vi "Untitled 1.vi"() -> ()   [LabVIEW 2014]
uses:
  <vilib>/userdefined/High Color/IMAQdx.ctl
  <vilib>/vision/Classification.llb/IMAQ Classifier Session.ctl
  <vilib>/vision/driver/NI_Vision_Acquisition_Software.lvlib
  <resource>/objmgr/imaqdx.rc
panel:
  out "Boolean":bool
  out "Classes (Color Classification 1)":string[](array[string])
  out "Classifier Session (Color Classification 1)":T1
  in  "video mode":u32
  out "processed":T2(plugin-control)
  out "source":T2(plugin-control)
  in  "ESC":bool
  out "frame rate [fps]":dbl(slide) scale=0.0..30.0
  out "error out":errorcluster
  in  "webcam":T3="cam0"
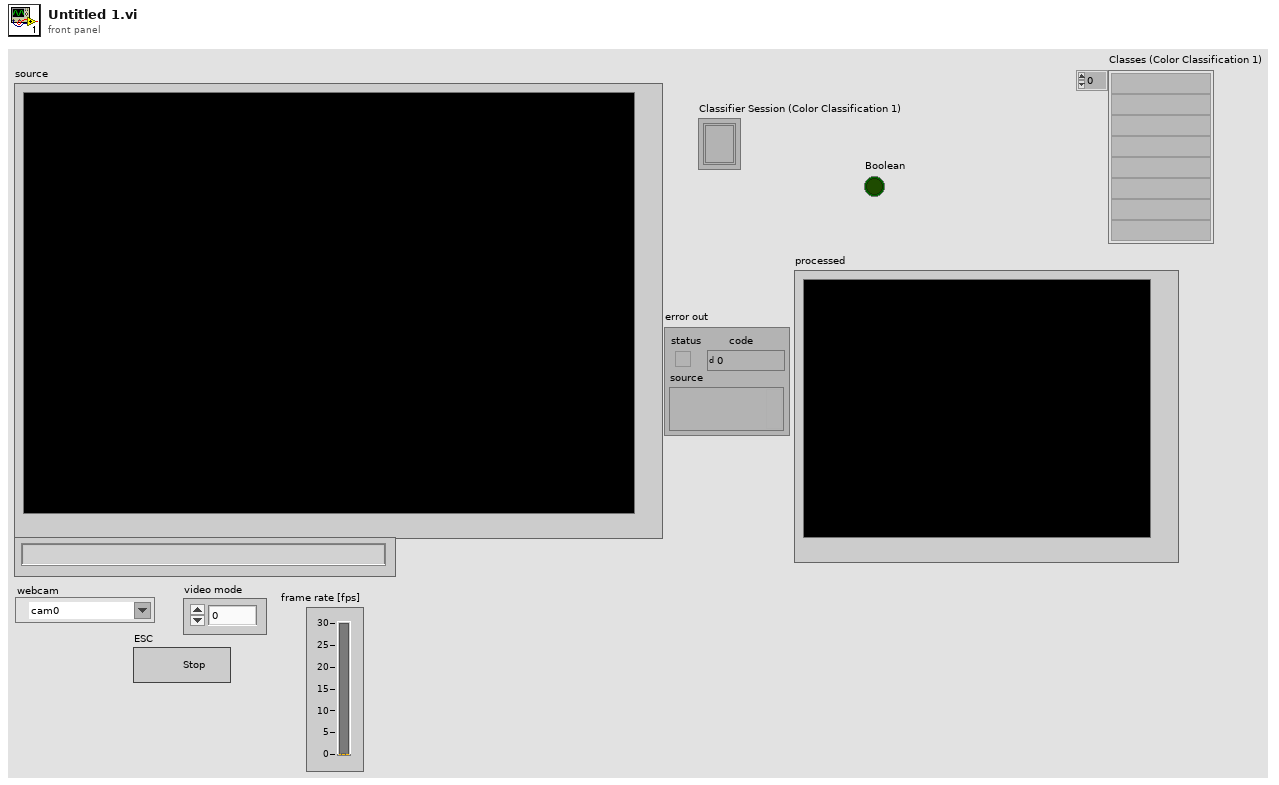
[diagram p1: front panel]
types:
  T1 = typedef "IMAQ Classifier Session.ctl" = refnum<k1>
  T2 = typedef "IMAQ Image.ctl" = refnum<image>
  T3 = typedef "IMAQdx.ctl" = refnum<k21>
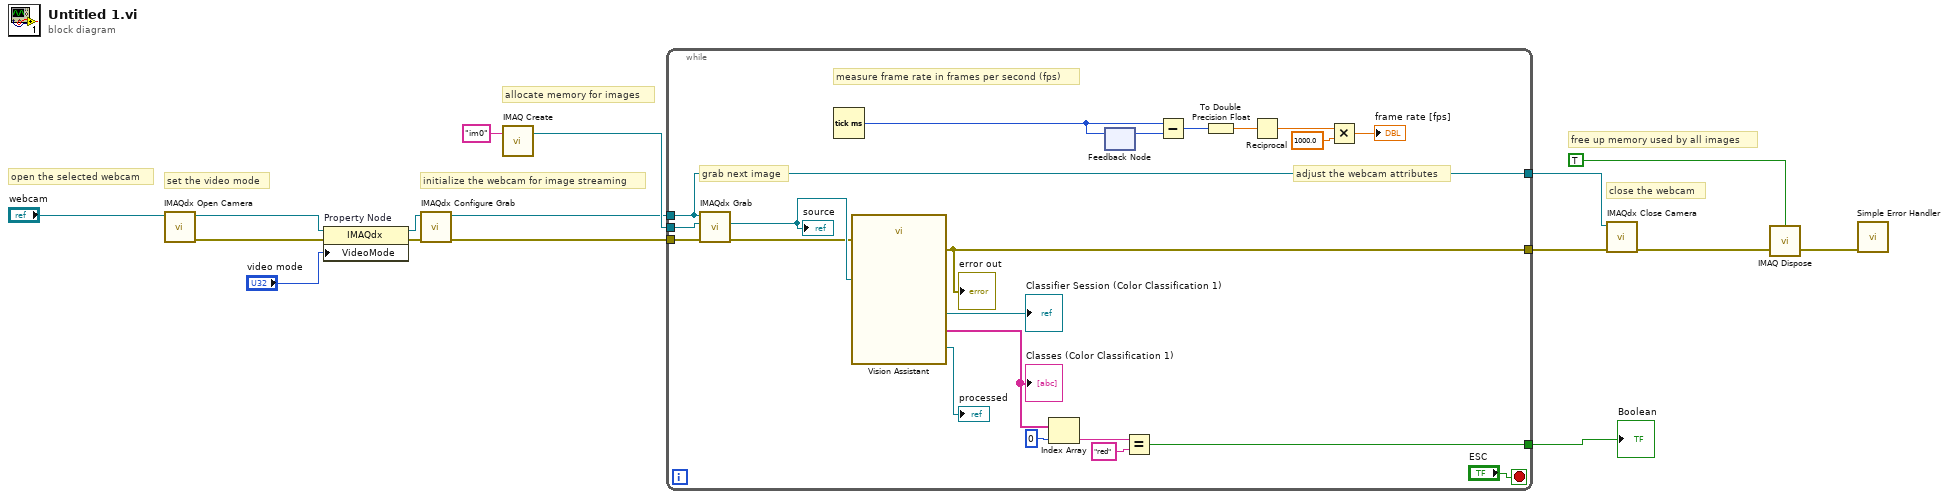
[diagram p0: block diagram]
diagram:
  # "close the webcam"
  # "open the selected webcam"
  # "set the video mode"
  # "allocate memory for images"
  # "initialize the webcam for image streaming"
  # "free up memory used by all images"
  n1 = call <vilib>:"IMAQdx Open Camera.vi"("Session In"="webcam") -> ("error out"=w7:errorcluster, "Session Out"=w6:T3)  [unwired: 2 in, 7 out]
  n2 = property on="Property Node" class="IMAQdx"(reference=w6, error in=w7, "VideoMode"="video mode") -> (reference out=w3:T3, error out=w4:errorcluster)
  n3 = call <vilib>:"IMAQdx Configure Grab.vi"("error in"=w4, "Session In"=w3) -> ("error out"=w13:errorcluster, "Session Out"=w8:T3)  [unwired: 8 in]
  n4 = call "IMAQ Create"("Image Name"="im0") -> ("New Image"=w14:T2)  [unwired: 3 in, 2 out]
  n5 = while {
    tunnel: w14 -> [w37]
    tunnel: w13 -> [w36]
    tunnel: w8 -> [w27]
    tunnel: [w27] -> w10
    tunnel: [w24] -> w2
    tunnel: [w17] -> w1
    stop <- "ESC" stop-if-true
    # "measure frame rate in frames per second (fps)"
    # "adjust the webcam attributes"
    # "grab next image"
    n6 = call <vilib>:"IMAQdx Grab.vi"("error in"=w36, "Image In"=w37, "Session In"=w27) -> ("error out"=w25:errorcluster, "Image Out"=w26:T2)  [unwired: 5 in, 2 out]
    "source" <- w26
    n7 = Tick Count (ms)() -> (millisecond timer value=w34:u32)
    n8 = call "Vision Assistant"("Image In"=w26, "error in"=w25) -> ("Image Out"=→"processed":T2, "Classifier Session (Color Classification 1)"=→"Classifier Session (Color Classification 1)":T1, "Classes (Color Classification 1)"=w20:string[], "error out"=w24:errorcluster)  [unwired: 22 in]
    "error out" <- w24
    "Classes (Color Classification 1)" <- w20
    n9 = Index Array(array=w20, index=0) -> (element=w19:string)
    n10 = feedback-in #1(w34) -> ()
    n11 = feedback #1() -> (w33:u32)  [unwired: 1 in]
    n12 = Equal?(x=w19, y="red") -> (x = y?=w17:bool)
    n13 = Subtract(x=w34, y=w33) -> (x-y=w32:u32)
    n14 = To Double Precision Float(number=w32) -> (double precision float=w31:dbl)
    n15 = Reciprocal(x=w31) -> (1/x=w30:dbl)
    n16 = Multiply(x=w30, y=1000.0) -> (x*y=→"frame rate [fps]":dbl)
  }
  "Boolean" <- w1
  n17 = call <vilib>:"IMAQdx Close Camera.vi"("error in"=w2, "Session In"=w10) -> ("error out"=w11:errorcluster)  [unwired: 9 out]
  n18 = call "IMAQ Dispose"("All Images? (No)"=TRUE, "error in (no error)"=w11) -> ("error out"=w9:errorcluster)  [unwired: 4 in]
  n19 = call <vilib>:"Simple Error Handler.vi"("error in (no error)"=w9) -> ()  [unwired: 4 in, 5 out]
